vi "main(TGA_DSC).vi"() -> ()   [LabVIEW 2011]
uses:
  subvi/dataType/TGA_DSC new data record.ctl
  subvi/dataType/TGA_DSC.ctl
panel:
  in  "停止":bool
  out "path":path
  out "passYeild":dbl=0.98
  out "DB":T1={"Server"="172.20.23.107", "DB"="MESDatacenter", "PSW"="data'songyy", "User"="sa"}
  out "DB2":T1={"Server"="172.20.23.107", "DB"="HTPSDB", "PSW"="data'songyy", "User"="sa"}
  out "uploadpath":path=path "d:/xmlconvert/upload"
  out "temppath":path=path "d:/xmlconvert/temp"
  out "successpath":path=path "d:/xmlconvert/success"
  out "failpath":path=path "d:/xmlconvert/fail"
  out "path":string="D:\\testzip"
  out "timeout":i32=10
  out "filter":string="*.zip"
  in  "start":bool caption="停止"
  out "状态:":string
  in  "exit":bool caption="停止"
  # "华为 Json生成器\nfor TGA,DSC,FTIR"
  # "Ver:1.00         20181126"
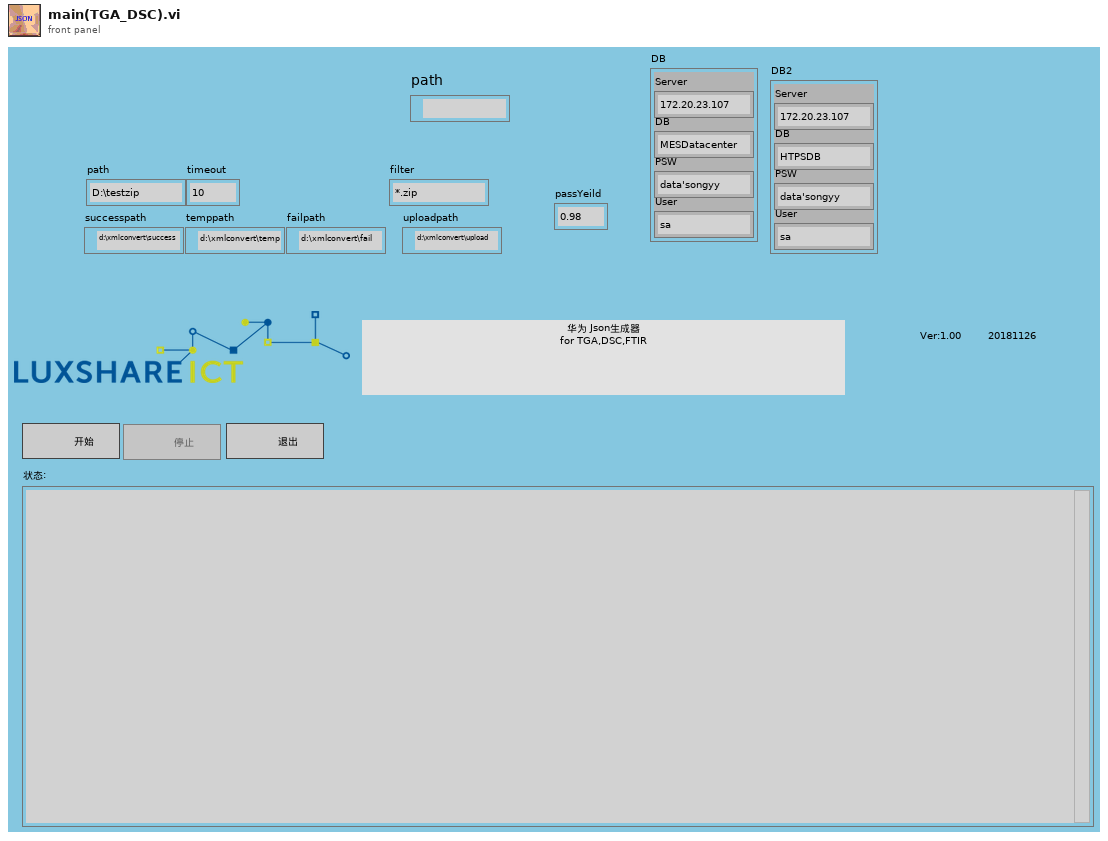
[diagram p1: front panel]
types:
  T1 = cluster{"Server":string, "DB":string, "PSW":string, "User":string}
  T2 = enum8{"Enabled", "Disabled", "Disabled and Grayed Out"}
  T3 = typedef "TGA_DSC new data record.ctl" = cluster{"id":string, "TGA/DSC":T4, "txtPath":path, "num":dbl, "lastone?":bool}
  T4 = typedef "TGA_DSC.ctl" = cluster{"materialCode":string, "SN":string, "pcName":string, "programmName":string, "startTime":string, "stopTime":string, "itemName":string}
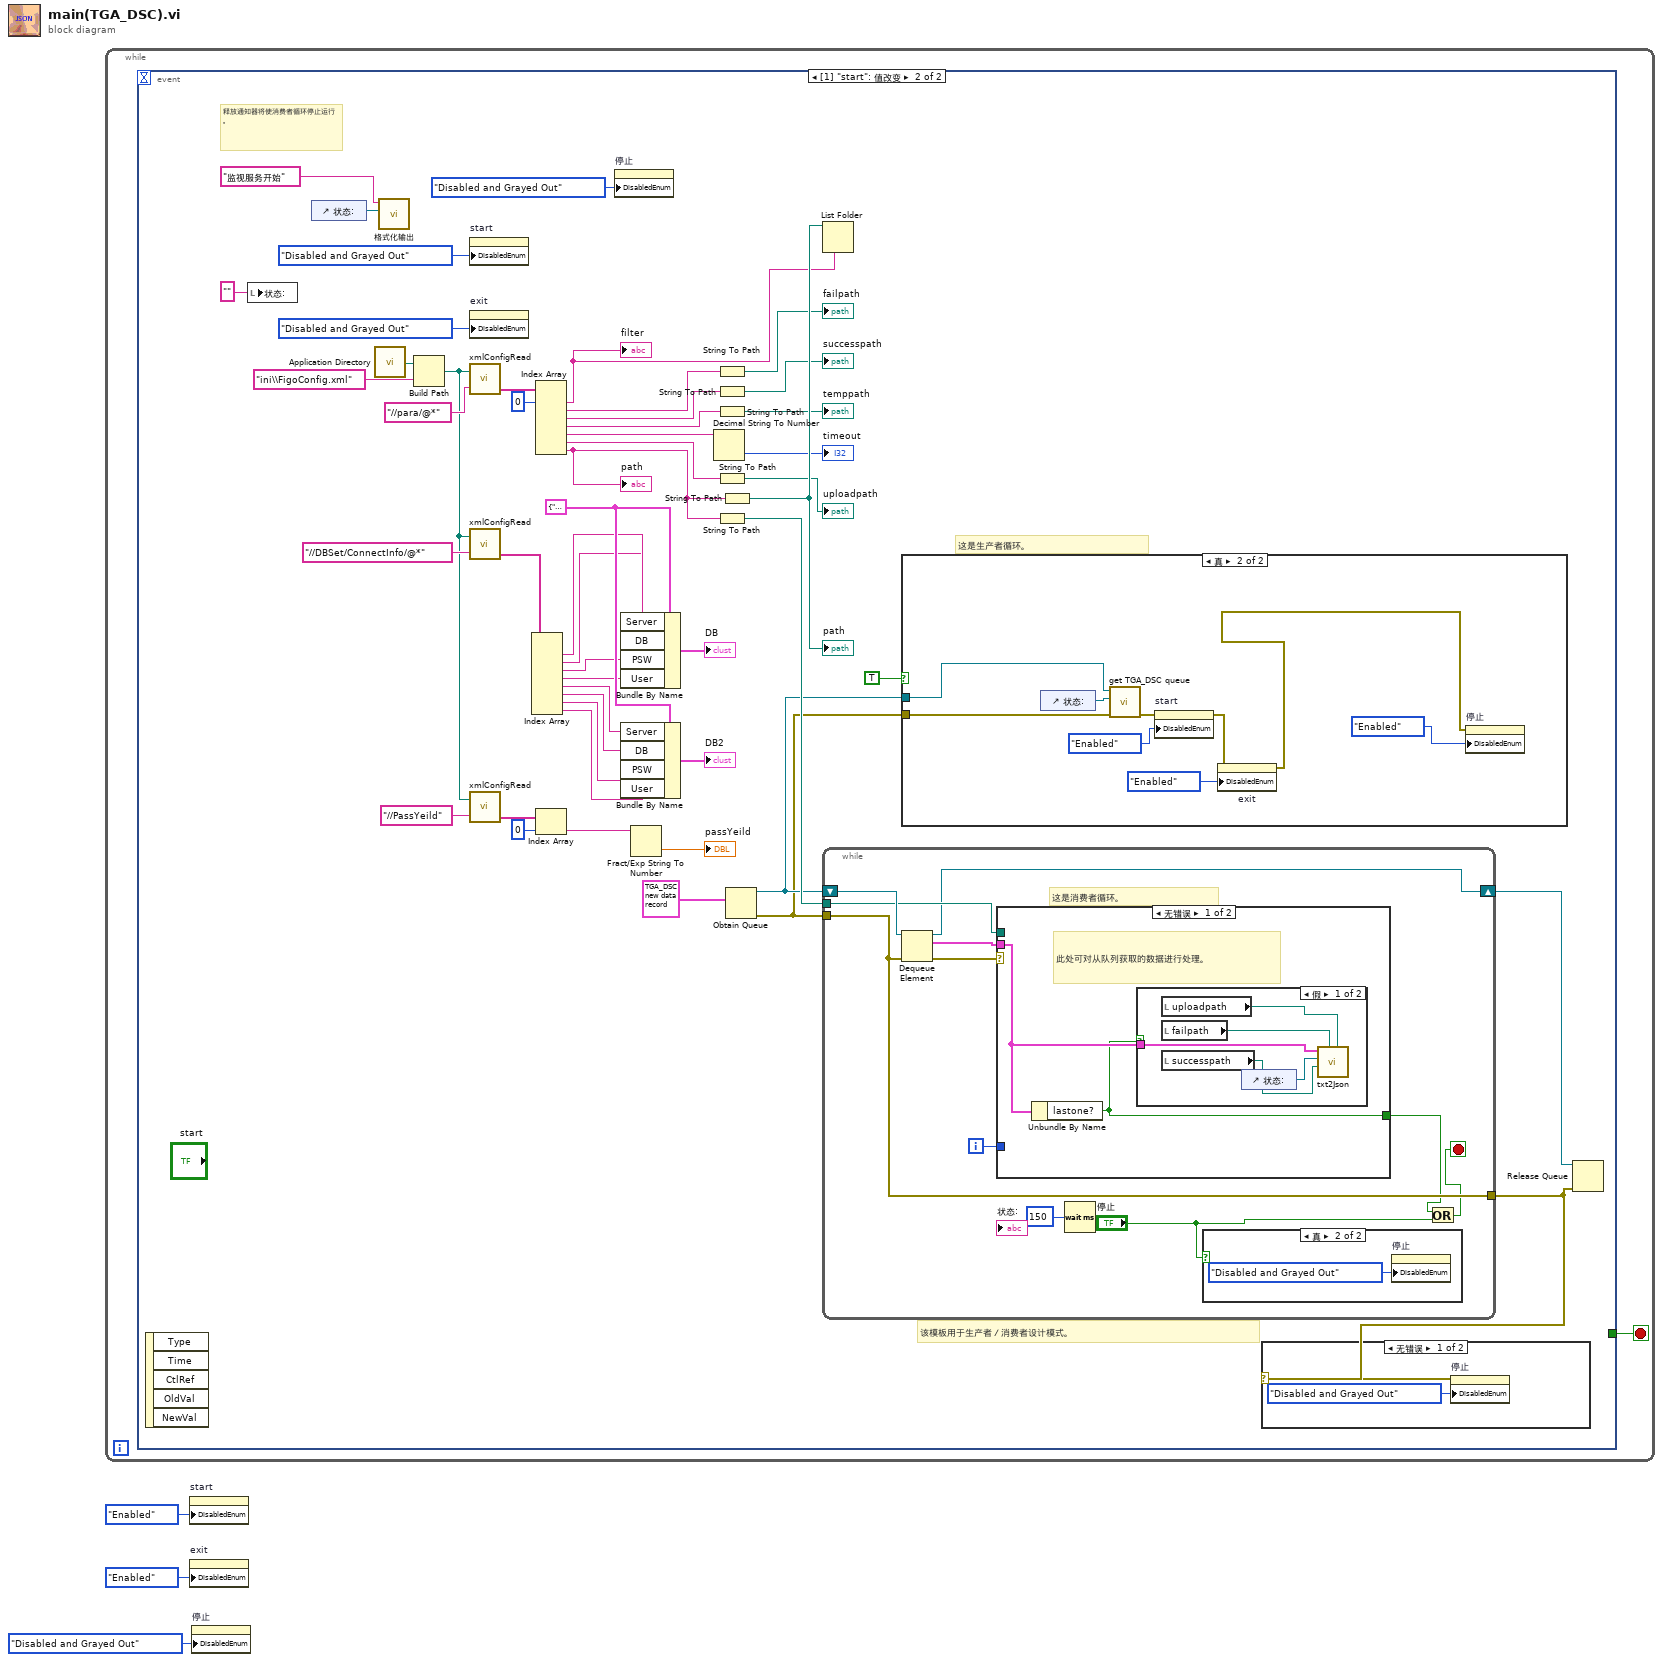
[diagram p0: block diagram]
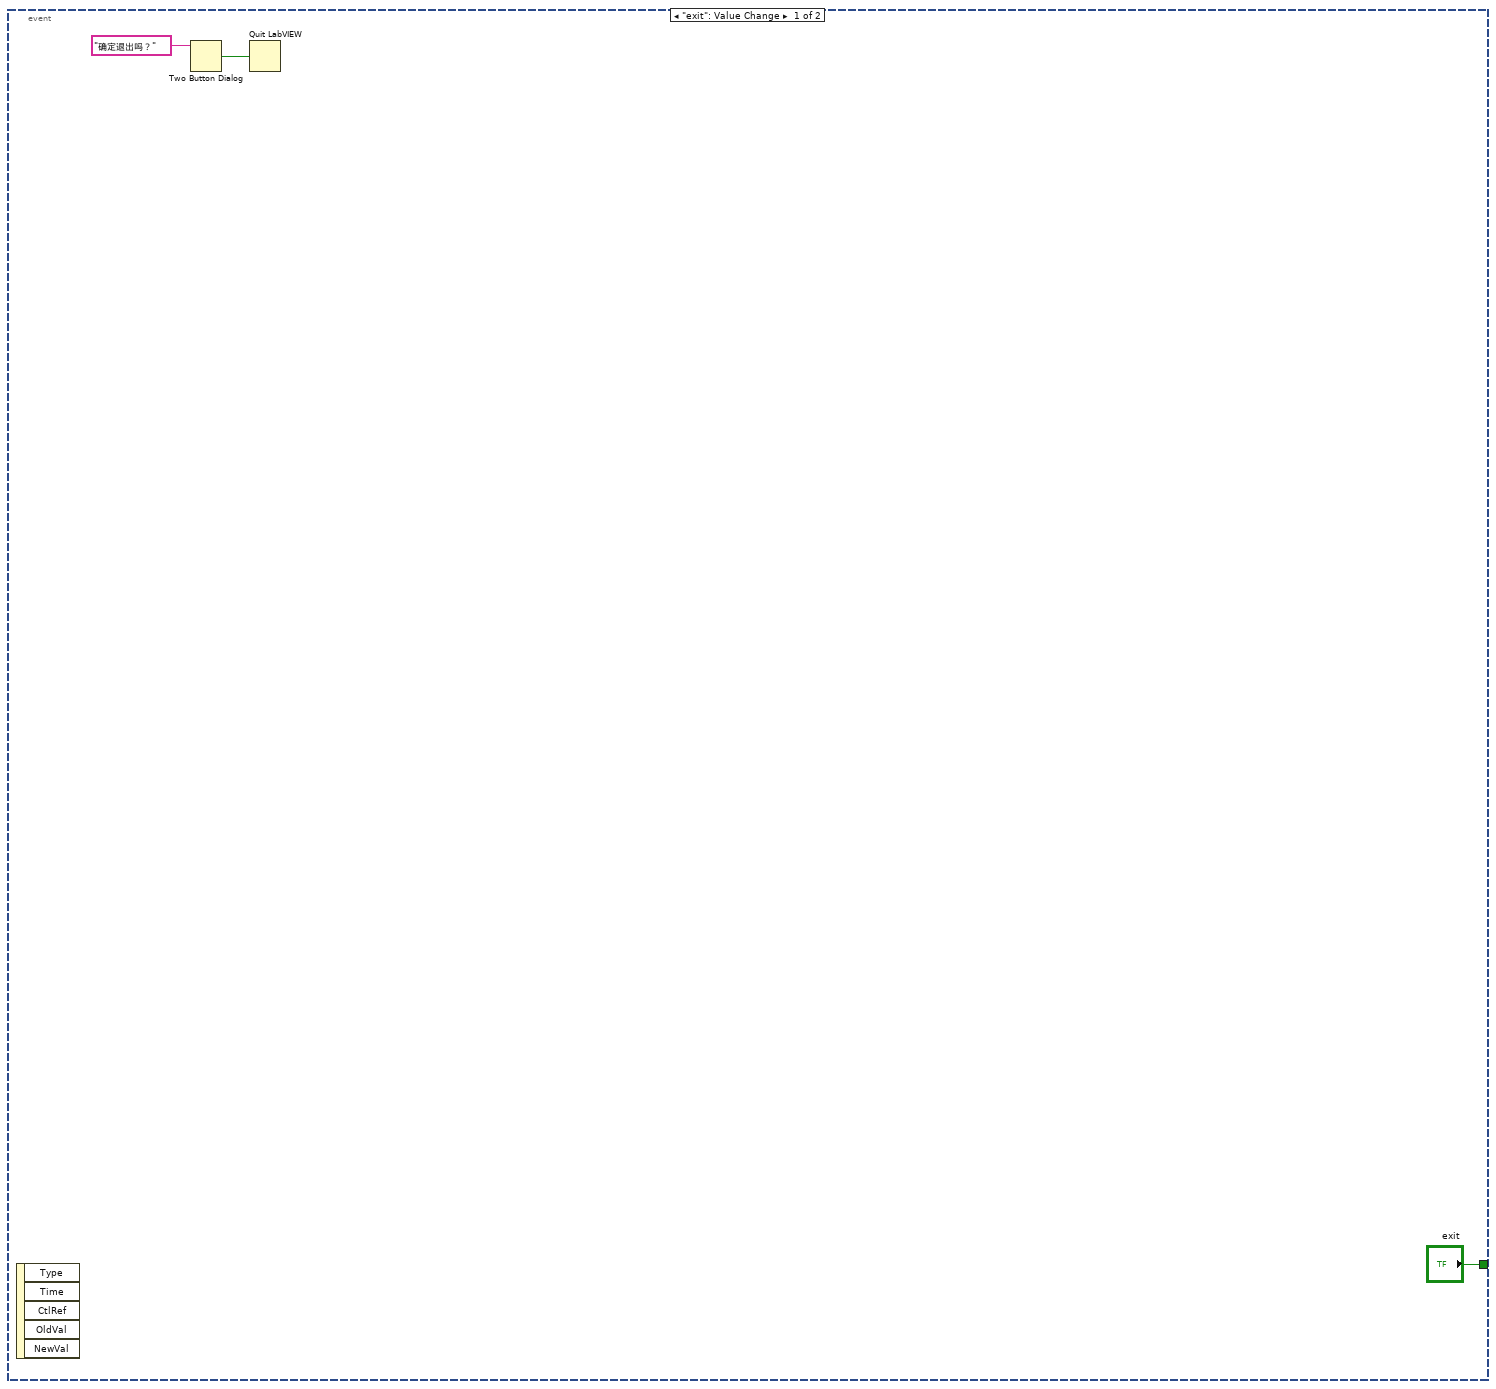
[diagram p2: hidden frame]
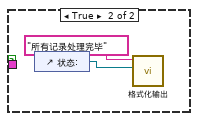
[diagram p6: hidden frame]
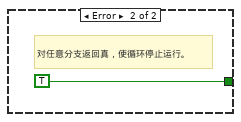
[diagram p7: hidden frame]
diagram:
  n1 = while {
    stop <- w4 stop-if-true
    n2 = event shown="[1] \"start\": 值改变" {
      selector: _ -> [_ _]
      dyn-events: _ -> [_ _]
      timeout: _ -> [_ _]
      tunnel: ["exit" _] -> w4
      event "exit": Value Change {
        n3 = event-data() -> ()  [unwired: 1 in, 5 out]
        n4 = Two Button Dialog(message="确定退出吗？" ("消息")) -> (T button?=w5:bool)  [unwired: 2 in]
        n5 = Quit LabVIEW(quit? (T)=w5) -> ()
      }
      event "start": Value Change {
        w31 = T1 {"Server"="", "DB"="", "PSW"="", "User"=""} ("DBSet")
        # "释放通知器将使消费者循环停止运行。"
        # "这是生产者循环。"
        # "该模板用于生产者／消费者设计模式。"
        n6 = event-data() -> ()  [unwired: 1 in, 5 out]
        n7 = local write "状态:"("" ("增加的文件")) -> ()
        n8 = control-ref of="状态:"() -> (w56:refnum<vi>)
        n9 = call <vilib>:"Application Directory.vi"() -> ("Application Directory"=w53:path)
        n10 = call "格式化输出.vi"("字符串引用"=w56, "字符串"="监视服务开始") -> ()  [unwired: 9 in, 1 out]
        n11 = Build Path(base path=w53, name or relative path="ini\\FigoConfig.xml" ("名称或相对路径")) -> (appended path=w19:path)
        n12 = property on="start" class="Bool"("DisabledEnum"=T2."Disabled and Grayed Out" ("禁用")) -> ()  [unwired: 2 in, 2 out]
        n13 = property on="exit" class="Bool"("DisabledEnum"=T2."Disabled and Grayed Out" ("禁用")) -> ()  [unwired: 2 in, 2 out]
        n14 = call "xmlConfigRead.vi"("path to XML document"=w19, "XPath expression"="//para/@*") -> ("OutParaArray"=w50:string[])  [unwired: 2 out]
        n15 = call "xmlConfigRead.vi"("path to XML document"=w19, "XPath expression"="//DBSet/ConnectInfo/@*") -> ("OutParaArray"=w32:string[])  [unwired: 2 out]
        n16 = call "xmlConfigRead.vi"("path to XML document"=w19, "XPath expression"="//PassYeild") -> ("OutParaArray"=w18:string[])  [unwired: 2 out]
        n17 = Index Array(array=w32) -> (element #1=w30:string, element #2=w29:string, element #3=w28:string, element #4=w27:string, element #5=w26:string, element #6=w25:string, element #7=w24:string, element #8=w23:string)  [unwired: 8 in]
        n18 = Index Array(array=w50, index #1=0 ("索引")) -> (element #1=w34:string, element #2=w45:string, element #3=w43:string, element #4=w40:string, element #5=w41:string, element #6=w38:string, element #7=w35:string)  [unwired: 6 in]
        "filter" <- w34
        "path" <- w35
        n19 = Index Array(array=w18, index=0 ("索引")) -> (element=w16:string)
        n20 = property on="停止" class="Bool"("DisabledEnum"=T2."Disabled and Grayed Out" ("禁用")) -> ()  [unwired: 2 in, 2 out]
        n21 = Bundle By Name(cluster=w31, "Server"=w30, "DB"=w29, "PSW"=w28, "User"=w27) -> (→"DB":T1)
        n22 = Bundle By Name(cluster=w31, "Server"=w26, "DB"=w25, "PSW"=w24, "User"=w23) -> (→"DB2":T1)
        n23 = Fract/Exp String To Number(string=w16) -> (number=→"passYeild":dbl)  [unwired: 3 in, 1 out]
        n24 = Decimal String To Number(string=w41) -> (number=→"timeout":i32)  [unwired: 2 in, 1 out]
        n25 = String To Path(string=w45) -> (path=→"failpath":path)
        n26 = String To Path(string=w43) -> (path=→"successpath":path)
        n27 = String To Path(string=w40) -> (path=→"temppath":path)
        n28 = String To Path(string=w38) -> (path=→"uploadpath":path)
        n29 = String To Path(string=w35) -> (path=w47:path)
        n30 = String To Path(string=w35) -> (path=w57:path)
        "path" <- w57
        n31 = Obtain Queue(element data type=T3 {"id"="", "TGA/DSC"={"materialCode"="", "SN"="", "pcName"="", "programmName"="", "startTime"="", "stopTime"="", "itemName"=""}, "txtPath"=path "", "num"=0.0, "lastone?"=FALSE} ("TGA/DSC new data")) -> (queue out=w13:refnum<queue>, error out=w11:errorcluster)  [unwired: 4 in, 1 out]
        n32 = List Folder(path=w57, pattern=w34) -> ()  [unwired: 2 in, 4 out]
        n33 = while {
          tunnel: w47 -> [w76]
          tunnel: w11 -> [w75]
          tunnel: [w75] -> w8
          shift-right: [w72] -> w10
          shift-left: w13 -> [w78]
          i -> [w73]
          stop <- w70 stop-if-true
          # "这是消费者循环。"
          n34 = Dequeue Element(queue=w78, error in (no error)=w75) -> (queue out=w72:refnum<queue>, element=w74:T3, error out=w79:errorcluster)  [unwired: 1 in, 1 out]
          n35 = case shown="无错误" w79 {
            tunnel: w74 -> [w82 _]
            tunnel: [w81 TRUE] -> w71
            tunnel: w76 -> [_ _]
            tunnel: w73 -> [_ _]
            frame No Error {
              # "此处可对从队列获取的数据进行处理。"
              n36 = Unbundle By Name(w82) -> ("lastone?"=w81:bool)
              n37 = case shown="假" w81 {
                tunnel: w82 -> [w83 _]
                frame False {
                  n38 = local read "uploadpath"() -> (w84:path)
                  n39 = local read "failpath"() -> (w85:path)
                  n40 = local read "successpath"() -> (w86:path)
                  n41 = control-ref of="状态:"() -> (w87:refnum<vi>)
                  n42 = call "txt2Json.vi"("uploadPath"=w84, "failpath"=w85, "successpath"=w86, "statusRef"=w87, "TGA/DSC new data"=w83) -> ()  [unwired: 6 in, 1 out]
                }
                frame True {
                  n43 = control-ref of="状态:"() -> (w89:refnum<vi>)
                  n44 = call "格式化输出.vi"("字符串引用"=w89, "字符串"="所有记录处理完毕") -> ()  [unwired: 9 in, 1 out]
                }
              }
            }
            frame Error {
              # "对任意分支返回真，使循环停止运行。"
            }
          }
          n45 = Wait (ms)(milliseconds to wait=u32 150 ("等待时间（毫秒）")) -> ()  [unwired: 1 out]
          n46 = case shown="真" "停止" {
            frame False {
            }
            frame True {
              n47 = property on="停止" class="Bool"("DisabledEnum"=T2."Disabled and Grayed Out" ("禁用")) -> ()  [unwired: 2 in, 2 out]
            }
          }
          n48 = Or(x=w71, y="停止") -> (x .or. y?=w70:bool)
        }
        n49 = case shown="真" TRUE ("Case Constant\n(See Context Help)") {
          tunnel: w13 -> [_ w68]
          tunnel: w11 -> [_ w67]
          frame False {
          }
          frame True {
            n50 = control-ref of="状态:"() -> (w66:refnum<vi>)
            n51 = call "get TGA_DSC queue.vi"("error in"=w67, "statusRef"=w66, "queue in"=w68) -> ("错误输出 2"=w64:errorcluster)  [unwired: 7 in, 1 out]
            n52 = property on="start" class="Bool"(error in=w64, "DisabledEnum"=T2."Enabled" ("禁用")) -> (error out=w62:errorcluster)  [unwired: 1 in, 1 out]
            n53 = property on="exit" class="Bool"(error in=w62, "DisabledEnum"=T2."Enabled" ("禁用")) -> (error out=w60:errorcluster)  [unwired: 1 in, 1 out]
            n54 = property on="停止" class="Bool"(error in=w60, "DisabledEnum"=T2."Enabled" ("禁用")) -> ()  [unwired: 1 in, 2 out]
          }
        }
        n55 = case shown="无错误" w8 {
          selector: w8 -> [w58 _]
          frame No Error {
            n56 = property on="停止" class="Bool"(error in=w58, "DisabledEnum"=T2."Disabled and Grayed Out" ("禁用")) -> ()  [unwired: 1 in, 2 out]
          }
          frame Error {
          }
        }
        n57 = Release Queue(queue=w10, error in (no error)=w8) -> ()  [unwired: 1 in, 3 out]
      }
    }
  }
  n58 = property on="start" class="Bool"("DisabledEnum"=T2."Enabled" ("禁用")) -> ()  [unwired: 2 in, 2 out]
  n59 = property on="exit" class="Bool"("DisabledEnum"=T2."Enabled" ("禁用")) -> ()  [unwired: 2 in, 2 out]
  n60 = property on="停止" class="Bool"("DisabledEnum"=T2."Disabled and Grayed Out" ("禁用")) -> ()  [unwired: 2 in, 2 out]
